vi "test TCX read (installed 71).vi"() -> ()   [LabVIEW 2011] (continued)
xmlns=\"http://www.garmin.com/xmlschemas/ActivityExtension/v2\"><Watts>208</Watts></TPX></Extensions></Trackpoint><Trackpoint><Time>2008-03-03T13:56:22Z</Time><Position><LatitudeDegrees>35.875378</LatitudeDegrees><LongitudeDegrees>-78.923548</LongitudeDegrees></Position><AltitudeMeters>77.523</AltitudeMeters><DistanceMeters>4523.565</DistanceMeters><Cadence>69</Cadence><Extensions><TPX xmlns=\"http://www.garmin.com/xmlschemas/ActivityExtension/v2\"><Watts>205</Watts></TPX></Extensions></Trackpoint><Trackpoint><Time>2008-03-03T13:56:23Z</Time><Position><LatitudeDegrees>35.875378</LatitudeDegrees><LongitudeDegrees>-78.923468</LongitudeDegrees></Position><AltitudeMeters>77.523</AltitudeMeters><DistanceMeters>4530.843</DistanceMeters><Cadence>68</Cadence><Extensions><TPX xmlns=\"http://www.garmin.com/xmlschemas/ActivityExtension/v2\"><Watts>201</Watts></TPX></Extensions></Trackpoint><Trackpoint><Time>2008-03-03T13:56:24Z</Time><Position><LatitudeDegrees>35.875380</LatitudeDegrees><LongitudeDegrees>-78.923390</LongitudeDegrees></Position><AltitudeMeters>77.523</AltitudeMeters><DistanceMeters>4537.809</DistanceMeters><Cadence>68</Cadence><Extensions><TPX xmlns=\"http://www.garmin.com/xmlschemas/ActivityExtension/v2\"><Watts>202</Watts></TPX></Extensions></Trackpoint><Trackpoint><Time>2008-03-03T13:56:25Z</Time><Position><LatitudeDegrees>35.875383</LatitudeDegrees><LongitudeDegrees>-78.923315</LongitudeDegrees></Position><AltitudeMeters>78.004</AltitudeMeters><DistanceMeters>4544.542</DistanceMeters><Cadence>68</Cadence><Extensions><TPX xmlns=\"http://www.garmin.com/xmlschemas/ActivityExtension/v2\"><Watts>207</Watts></TPX></Extensions></Trackpoint><Trackpoint><Time>2008-03-03T13:56:26Z</Time><Position><LatitudeDegrees>35.875382</LatitudeDegrees><LongitudeDegrees>-78.923243</LongitudeDegrees></Position><AltitudeMeters>78.485</AltitudeMeters><DistanceMeters>4551.062</DistanceMeters><Cadence>67</Cadence><Extensions><TPX xmlns=\"http://www.garmin.com/xmlschemas/ActivityExtension/v2\"><Watts>264</Watts></TPX></Extensions></Trackpoint><Trackpoint><Time>2008-03-03T13:56:27Z</Time><Position><LatitudeDegrees>35.875381</LatitudeDegrees><LongitudeDegrees>-78.923173</LongitudeDegrees></Position><AltitudeMeters>78.965</AltitudeMeters><DistanceMeters>4557.379</DistanceMeters><Cadence>69</Cadence><Extensions><TPX xmlns=\"http://www.garmin.com/xmlschemas/ActivityExtension/v2\"><Watts>374</Watts></TPX></Extensions></Trackpoint><Trackpoint><Time>2008-03-03T13:56:28Z</Time><Position><LatitudeDegrees>35.875390</LatitudeDegrees><LongitudeDegrees>-78.923102</LongitudeDegrees></Position><AltitudeMeters>78.965</AltitudeMeters><DistanceMeters>4563.882</DistanceMeters><Cadence>70</Cadence><Extensions><TPX xmlns=\"http://www.garmin.com/xmlschemas/ActivityExtension/v2\"><Watts>494</Watts></TPX></Extensions></Trackpoint><Trackpoint><Time>2008-03-03T13:56:29Z</Time><Position><LatitudeDegrees>35.875391</LatitudeDegrees><LongitudeDegrees>-78.923028</LongitudeDegrees></Position><AltitudeMeters>79.446</AltitudeMeters><DistanceMeters>4570.581</DistanceMeters><Cadence>70</Cadence><Extensions><TPX xmlns=\"http://www.garmin.com/xmlschemas/ActivityExtension/v2\"><Watts>505</Watts></TPX></Extensions></Trackpoint><Trackpoint><Time>2008-03-03T13:56:30Z</Time><Position><LatitudeDegrees>35.875391</LatitudeDegrees><LongitudeDegrees>-78.922954</LongitudeDegrees></Position><AltitudeMeters>80.407</AltitudeMeters><DistanceMeters>4577.208</DistanceMeters><Cadence>70</Cadence><Extensions><TPX xmlns=\"http://www.garmin.com/xmlschemas/ActivityExtension/v2\"><Watts>564</Watts></TPX></Extensions></Trackpoint><Trackpoint><Time>2008-03-03T13:56:31Z</Time><Position><LatitudeDegrees>35.875394</LatitudeDegrees><LongitudeDegrees>-78.922883</LongitudeDegrees></Position><AltitudeMeters>80.407</AltitudeMeters><DistanceMeters>4583.685</DistanceMeters><Cadence>70</Cadence><Extensions><TPX xmlns=\"http://www.garmin.com/xmlschemas/ActivityExtension/v2\"><Watts>578</Watts></TPX></Extensions></Trackpoint><Trackpoint><Time>2008-03-03T13:56:32Z</Time><Position><LatitudeDegrees>35.875403</LatitudeDegrees><LongitudeDegrees>-78.922812</LongitudeDegrees></Position><AltitudeMeters>80.888</AltitudeMeters><DistanceMeters>4590.137</DistanceMeters><Cadence>68</Cadence><Extensions><TPX xmlns=\"http://www.garmin.com/xmlschemas/ActivityExtension/v2\"><Watts>569</Watts></TPX></Extensions></Trackpoint><Trackpoint><Time>2008-03-03T13:56:33Z</Time><Position><LatitudeDegrees>35.875404</LatitudeDegrees><LongitudeDegrees>-78.922740</LongitudeDegrees></Position><AltitudeMeters>81.849</AltitudeMeters><DistanceMeters>4596.551</DistanceMeters><Cadence>67</Cadence><Extensions><TPX xmlns=\"http://www.garmin.com/xmlschemas/ActivityExtension/v2\"><Watts>513</Watts></TPX></Extensions></Trackpoint><Trackpoint><Time>2008-03-03T13:56:34Z</Time><Position><LatitudeDegrees>35.875407</LatitudeDegrees><LongitudeDegrees>-78.922669</LongitudeDegrees></Position><AltitudeMeters>82.811</AltitudeMeters><DistanceMeters>4602.985</DistanceMeters><Cadence>67</Cadence><Extensions><TPX xmlns=\"http://www.garmin.com/xmlschemas/ActivityExtension/v2\"><Watts>512</Watts></TPX></Extensions></Trackpoint><Trackpoint><Time>2008-03-03T13:56:35Z</Time><Position><LatitudeDegrees>35.875412</LatitudeDegrees><LongitudeDegrees>-78.922599</LongitudeDegrees></Position><AltitudeMeters>82.330</AltitudeMeters><DistanceMeters>4609.317</DistanceMeters><Cadence>68</Cadence><Extensions><TPX xmlns=\"http://www.garmin.com/xmlschemas/ActivityExtension/v2\"><Watts>434</Watts></TPX></Extensions></Trackpoint><Trackpoint><Time>2008-03-03T13:56:36Z</Time><Position><LatitudeDegrees>35.875413</LatitudeDegrees><LongitudeDegrees>-78.922528</LongitudeDegrees></Position><AltitudeMeters>82.811</AltitudeMeters><DistanceMeters>4615.766</DistanceMeters><Cadence>70</Cadence><Extensions><TPX xmlns=\"http://www.garmin.com/xmlschemas/ActivityExtension/v2\"><Watts>394</Watts></TPX></Extensions></Trackpoint><Trackpoint><Time>2008-03-03T13:56:37Z</Time><Position><LatitudeDegrees>35.875414</LatitudeDegrees><LongitudeDegrees>-78.922452</LongitudeDegrees></Position><AltitudeMeters>82.330</AltitudeMeters><DistanceMeters>4622.678</DistanceMeters><Cadence>72</Cadence><Extensions><TPX xmlns=\"http://www.garmin.com/xmlschemas/ActivityExtension/v2\"><Watts>358</Watts></TPX></Extensions></Trackpoint><Trackpoint><Time>2008-03-03T13:56:38Z</Time><Position><LatitudeDegrees>35.875414</LatitudeDegrees><LongitudeDegrees>-78.922373</LongitudeDegrees></Position><AltitudeMeters>82.811</AltitudeMeters><DistanceMeters>4629.848</DistanceMeters><Cadence>75</Cadence><Extensions><TPX xmlns=\"http://www.garmin.com/xmlschemas/ActivityExtension/v2\"><Watts>320</Watts></TPX></Extensions></Trackpoint><Trackpoint><Time>2008-03-03T13:56:39Z</Time><Position><LatitudeDegrees>35.875413</LatitudeDegrees><LongitudeDegrees>-78.922292</LongitudeDegrees></Position><AltitudeMeters>82.330</AltitudeMeters><DistanceMeters>4637.147</DistanceMeters><Cadence>75</Cadence><Extensions><TPX xmlns=\"http://www.garmin.com/xmlschemas/ActivityExtension/v2\"><Watts>321</Watts></TPX></Extensions></Trackpoint><Trackpoint><Time>2008-03-03T13:56:40Z</Time><Position><LatitudeDegrees>35.875414</LatitudeDegrees><LongitudeDegrees>-78.922211</LongitudeDegrees></Position><AltitudeMeters>82.330</AltitudeMeters><DistanceMeters>4644.467</DistanceMeters><Cadence>75</Cadence><Extensions><TPX xmlns=\"http://www.garmin.com/xmlschemas/ActivityExtension/v2\"><Watts>135</Watts></TPX></Extensions></Trackpoint><Trackpoint><Time>2008-03-03T13:56:41Z</Time><Position><LatitudeDegrees>35.875416</LatitudeDegrees><LongitudeDegrees>-78.922128</LongitudeDegrees></Position><AltitudeMeters>82.811</AltitudeMeters><DistanceMeters>4651.992</DistanceMeters><Cadence>69</Cadence><Extensions><TPX xmlns=\"http://www.garmin.com/xmlschemas/ActivityExtension/v2\"><Watts>125</Watts></TPX></Extensions></Trackpoint><Trackpoint><Time>2008-03-03T13:56:42Z</Time><Position><LatitudeDegrees>35.875415</LatitudeDegrees><LongitudeDegrees>-78.922042</LongitudeDegrees></Position><AltitudeMeters>82.330</AltitudeMeters><DistanceMeters>4659.760</DistanceMeters><Cadence>71</Cadence><Extensions><TPX xmlns=\"http://www.garmin.com/xmlschemas/ActivityExtension/v2\"><Watts>114</Watts></TPX></Extensions></Trackpoint><Trackpoint><Time>2008-03-03T13:56:43Z</Time><Position><LatitudeDegrees>35.875410</LatitudeDegrees><LongitudeDegrees>-78.921953</LongitudeDegrees></Position><AltitudeMeters>82.330</AltitudeMeters><DistanceMeters>4667.842</DistanceMeters><Cadence>69</Cadence><Extensions><TPX xmlns=\"http://www.garmin.com/xmlschemas/ActivityExtension/v2\"><Watts>102</Watts></TPX></Extensions></Trackpoint><Trackpoint><Time>2008-03-03T13:56:44Z</Time><Position><LatitudeDegrees>35.875404</LatitudeDegrees><LongitudeDegrees>-78.921860</LongitudeDegrees></Position><AltitudeMeters>81.849</AltitudeMeters><DistanceMeters>4676.255</DistanceMeters><Cadence>69</Cadence><Extensions><TPX xmlns=\"http://www.garmin.com/xmlschemas/ActivityExtension/v2\"><Watts>89</Watts></TPX></Extensions></Trackpoint><Trackpoint><Time>2008-03-03T13:56:45Z</Time><Position><LatitudeDegrees>35.875404</LatitudeDegrees><LongitudeDegrees>-78.921764</LongitudeDegrees></Position><AltitudeMeters>80.888</AltitudeMeters><DistanceMeters>4684.944</DistanceMeters><Cadence>67</Cadence><Extensions><TPX xmlns=\"http://www.garmin.com/xmlschemas/ActivityExtension/v2\"><Watts>90</Watts></TPX></Extensions></Trackpoint><Trackpoint><Time>2008-03-03T13:56:46Z</Time><Position><LatitudeDegrees>35.875404</LatitudeDegrees><LongitudeDegrees>-78.921664</LongitudeDegrees></Position><AltitudeMeters>80.888</AltitudeMeters><DistanceMeters>4693.956</DistanceMeters><Cadence>68</Cadence><Extensions><TPX xmlns=\"http://www.garmin.com/xmlschemas/ActivityExtension/v2\"><Watts>110</Watts></TPX></Extensions></Trackpoint><Trackpoint><Time>2008-03-03T13:56:47Z</Time><Position><LatitudeDegrees>35.875406</LatitudeDegrees><LongitudeDegrees>-78.921562</LongitudeDegrees></Position><AltitudeMeters>80.888</AltitudeMeters><DistanceMeters>4703.153</DistanceMeters><Cadence>70</Cadence><Extensions><TPX xmlns=\"http://www.garmin.com/xmlschemas/ActivityExtension/v2\"><Watts>137</Watts></TPX></Extensions></Trackpoint><Trackpoint><Time>2008-03-03T13:56:48Z</Time><Position><LatitudeDegrees>35.875412</LatitudeDegrees><LongitudeDegrees>-78.921459</LongitudeDegrees></Position><AltitudeMeters>80.407</AltitudeMeters><DistanceMeters>4712.552</DistanceMeters><Cadence>71</Cadence><Extensions><TPX xmlns=\"http://www.garmin.com/xmlschemas/ActivityExtension/v2\"><Watts>156</Watts></TPX></Extensions></Trackpoint><Trackpoint><Time>2008-03-03T13:56:49Z</Time><Position><LatitudeDegrees>35.875417</LatitudeDegrees><LongitudeDegrees>-78.921355</LongitudeDegrees></Position><AltitudeMeters>80.407</AltitudeMeters><DistanceMeters>4721.973</DistanceMeters><Cadence>71</Cadence><Extensions><TPX xmlns=\"http://www.garmin.com/xmlschemas/ActivityExtension/v2\"><Watts>177</Watts></TPX></Extensions></Trackpoint><Trackpoint><Time>2008-03-03T13:56:50Z</Time><Position><LatitudeDegrees>35.875419</LatitudeDegrees><LongitudeDegrees>-78.921249</LongitudeDegrees></Position><AltitudeMeters>79.927</AltitudeMeters><DistanceMeters>4731.501</DistanceMeters><Cadence>72</Cadence><Extensions><TPX xmlns=\"http://www.garmin.com/xmlschemas/ActivityExtension/v2\"><Watts>205</Watts></TPX></Extensions></Trackpoint><Trackpoint><Time>2008-03-03T13:56:51Z</Time><Position><LatitudeDegrees>35.875421</LatitudeDegrees><LongitudeDegrees>-78.921144</LongitudeDegrees></Position><AltitudeMeters>80.407</AltitudeMeters><DistanceMeters>4741.016</DistanceMeters><Cadence>72</Cadence><Extensions><TPX xmlns=\"http://www.garmin.com/xmlschemas/ActivityExtension/v2\"><Watts>204</Watts></TPX></Extensions></Trackpoint><Trackpoint><Time>2008-03-03T13:56:52Z</Time><Position><LatitudeDegrees>35.875422</LatitudeDegrees><LongitudeDegrees>-78.921038</LongitudeDegrees></Position><AltitudeMeters>80.407</AltitudeMeters><DistanceMeters>4750.605</DistanceMeters><Cadence>72</Cadence><Extensions><TPX xmlns=\"http://www.garmin.com/xmlschemas/ActivityExtension/v2\"><Watts>223</Watts></TPX></Extensions></Trackpoint><Trackpoint><Time>2008-03-03T13:56:53Z</Time><Position><LatitudeDegrees>35.875425</LatitudeDegrees><LongitudeDegrees>-78.920933</LongitudeDegrees></Position><AltitudeMeters>79.927</AltitudeMeters><DistanceMeters>4760.038</DistanceMeters><Cadence>72</Cadence><Extensions><TPX xmlns=\"http://www.garmin.com/xmlschemas/ActivityExtension/v2\"><Watts>226</Watts></TPX></Extensions></Trackpoint><Trackpoint><Time>2008-03-03T13:56:54Z</Time><Position><LatitudeDegrees>35.875429</LatitudeDegrees><LongitudeDegrees>-78.920829</LongitudeDegrees></Position><AltitudeMeters>80.407</AltitudeMeters><DistanceMeters>4769.412</DistanceMeters><Cadence>71</Cadence><Extensions><TPX xmlns=\"http://www.garmin.com/xmlschemas/ActivityExtension/v2\"><Watts>202</Watts></TPX></Extensions></Trackpoint><Trackpoint><Time>2008-03-03T13:56:55Z</Time><Position><LatitudeDegrees>35.875434</LatitudeDegrees><LongitudeDegrees>-78.920726</LongitudeDegrees></Position><AltitudeMeters>79.927</AltitudeMeters><DistanceMeters>4778.739</DistanceMeters><Cadence>71</Cadence><Extensions><TPX xmlns=\"http://www.garmin.com/xmlschemas/ActivityExtension/v2\"><Watts>165</Watts></TPX></Extensions></Trackpoint><Trackpoint><Time>2008-03-03T13:56:56Z</Time><Position><LatitudeDegrees>35.875437</LatitudeDegrees><LongitudeDegrees>-78.920622</LongitudeDegrees></Position><AltitudeMeters>79.927</AltitudeMeters><DistanceMeters>4788.193</DistanceMeters><Cadence>71</Cadence><Extensions><TPX xmlns=\"http://www.garmin.com/xmlschemas/ActivityExtension/v2\"><Watts>163</Watts></TPX></Extensions></Trackpoint><Trackpoint><Time>2008-03-03T13:56:57Z</Time><Position><LatitudeDegrees>35.875439</LatitudeDegrees><LongitudeDegrees>-78.920514</LongitudeDegrees></Position><AltitudeMeters>79.927</AltitudeMeters><DistanceMeters>4797.911</DistanceMeters><Cadence>74</Cadence><Extensions><TPX xmlns=\"http://www.garmin.com/xmlschemas/ActivityExtension/v2\"><Watts>116</Watts></TPX></Extensions></Trackpoint><Trackpoint><Time>2008-03-03T13:56:58Z</Time><Position><LatitudeDegrees>35.875442</LatitudeDegrees><LongitudeDegrees>-78.920403</LongitudeDegrees></Position><AltitudeMeters>78.965</AltitudeMeters><DistanceMeters>4807.962</DistanceMeters><Cadence>76</Cadence><Extensions><TPX xmlns=\"http://www.garmin.com/xmlschemas/ActivityExtension/v2\"><Watts>108</Watts></TPX></Extensions></Trackpoint><Trackpoint><Time>2008-03-03T13:56:59Z</Time><Position><LatitudeDegrees>35.875448</LatitudeDegrees><LongitudeDegrees>-78.920288</LongitudeDegrees></Position><AltitudeMeters>79.446</AltitudeMeters><DistanceMeters>4818.466</DistanceMeters><Cadence>79</Cadence><Extensions><TPX xmlns=\"http://www.garmin.com/xmlschemas/ActivityExtension/v2\"><Watts>108</Watts></TPX></Extensions></Trackpoint><Trackpoint><Time>2008-03-03T13:57:00Z</Time><Position><LatitudeDegrees>35.875454</LatitudeDegrees><LongitudeDegrees>-78.920167</LongitudeDegrees></Position><AltitudeMeters>78.485</AltitudeMeters><DistanceMeters>4829.355</DistanceMeters><Cadence>84</Cadence><Extensions><TPX xmlns=\"http://www.garmin.com/xmlschemas/ActivityExtension/v2\"><Watts>102</Watts></TPX></Extensions></Trackpoint><Trackpoint><Time>2008-03-03T13:57:01Z</Time><Position><LatitudeDegrees>35.875459</LatitudeDegrees><LongitudeDegrees>-78.920043</LongitudeDegrees></Position><AltitudeMeters>78.004</AltitudeMeters><DistanceMeters>4840.638</DistanceMeters><Cadence>85</Cadence><Extensions><TPX xmlns=\"http://www.garmin.com/xmlschemas/ActivityExtension/v2\"><Watts>100</Watts></TPX></Extensions></Trackpoint><Trackpoint><Time>2008-03-03T13:57:02Z</Time><Position><LatitudeDegrees>35.875466</LatitudeDegrees><LongitudeDegrees>-78.919916</LongitudeDegrees></Position><AltitudeMeters>77.043</AltitudeMeters><DistanceMeters>4852.169</DistanceMeters><Cadence>87</Cadence><Extensions><TPX xmlns=\"http://www.garmin.com/xmlschemas/ActivityExtension/v2\"><Watts>102</Watts></TPX></Extensions></Trackpoint><Trackpoint><Time>2008-03-03T13:57:03Z</Time><Position><LatitudeDegrees>35.875471</LatitudeDegrees><LongitudeDegrees>-78.919786</LongitudeDegrees></Position><AltitudeMeters>76.562</AltitudeMeters><DistanceMeters>4863.915</DistanceMeters><Cadence>89</Cadence><Extensions><TPX xmlns=\"http://www.garmin.com/xmlschemas/ActivityExtension/v2\"><Watts>106</Watts></TPX></Extensions></Trackpoint><Trackpoint><Time>2008-03-03T13:57:04Z</Time><Position><LatitudeDegrees>35.875501</LatitudeDegrees><LongitudeDegrees>-78.919659</LongitudeDegrees></Position><AltitudeMeters>76.562</AltitudeMeters><DistanceMeters>4875.472</DistanceMeters><Cadence>90</Cadence><Extensions><TPX xmlns=\"http://www.garmin.com/xmlschemas/ActivityExtension/v2\"><Watts>120</Watts></TPX></Extensions></Trackpoint><Trackpoint><Time>2008-03-03T13:57:05Z</Time><Position><LatitudeDegrees>35.875514</LatitudeDegrees><LongitudeDegrees>-78.919528</LongitudeDegrees></Position><AltitudeMeters>76.562</AltitudeMeters><DistanceMeters>4887.392</DistanceMeters><Cadence>92</Cadence><Extensions><TPX xmlns=\"http://www.garmin.com/xmlschemas/ActivityExtension/v2\"><Watts>196</Watts></TPX></Extensions></Trackpoint><Trackpoint><Time>2008-03-03T13:57:06Z</Time><Position><LatitudeDegrees>35.875526</LatitudeDegrees><LongitudeDegrees>-78.919395</LongitudeDegrees></Position><AltitudeMeters>75.120</AltitudeMeters><DistanceMeters>4899.475</DistanceMeters><Cadence>92</Cadence><Extensions><TPX xmlns=\"http://www.garmin.com/xmlschemas/ActivityExtension/v2\"><Watts>194</Watts></TPX></Extensions></Trackpoint><Trackpoint><Time>2008-03-03T13:57:07Z</Time><Position><LatitudeDegrees>35.875539</LatitudeDegrees><LongitudeDegrees>-78.919260</LongitudeDegrees></Position><AltitudeMeters>74.640</AltitudeMeters><DistanceMeters>4911.710</DistanceMeters><Cadence>92</Cadence><Extensions><TPX xmlns=\"http://www.garmin.com/xmlschemas/ActivityExtension/v2\"><Watts>168</Watts></TPX></Extensions></Trackpoint><Trackpoint><Time>2008-03-03T13:57:08Z</Time><Position><LatitudeDegrees>35.875557</LatitudeDegrees><LongitudeDegrees>-78.919127</LongitudeDegrees></Position><AltitudeMeters>75.120</AltitudeMeters><DistanceMeters>4923.924</DistanceMeters><Cadence>92</Cadence><Extensions><TPX xmlns=\"http://www.garmin.com/xmlschemas/ActivityExtension/v2\"><Watts>167</Watts></TPX></Extensions></Trackpoint><Trackpoint><Time>2008-03-03T13:57:09Z</Time><Position><LatitudeDegrees>35.875570</LatitudeDegrees><LongitudeDegrees>-78.918995</LongitudeDegrees></Position><AltitudeMeters>74.640</AltitudeMeters><DistanceMeters>4935.932</DistanceMeters><Cadence>91</Cadence><Extensions><TPX xmlns=\"http://www.garmin.com/xmlschemas/ActivityExtension/v2\"><Watts>131</Watts></TPX></Extensions></Trackpoint><Trackpoint><Time>2008-03-03T13:57:10Z</Time><Position><LatitudeDegrees>35.875582</LatitudeDegrees><LongitudeDegrees>-78.918863</LongitudeDegrees></Position><AltitudeMeters>74.159</AltitudeMeters><DistanceMeters>4947.869</DistanceMeters><Cadence>90</Cadence><Extensions><TPX xmlns=\"http://www.garmin.com/xmlschemas/ActivityExtension/v2\"><Watts>131</Watts></TPX></Extensions></Trackpoint><Trackpoint><Time>2008-03-03T13:57:11Z</Time><Position><LatitudeDegrees>35.875593</LatitudeDegrees><LongitudeDegrees>-78.918733</LongitudeDegrees></Position><AltitudeMeters>74.159</AltitudeMeters><DistanceMeters>4959.708</DistanceMeters><Cadence>90</Cadence><Extensions><TPX xmlns=\"http://www.garmin.com/xmlschemas/ActivityExtension/v2\"><Watts>133</Watts></TPX></Extensions></Trackpoint><Trackpoint><Time>2008-03-03T13:57:12Z</Time><Position><LatitudeDegrees>35.875601</LatitudeDegrees><LongitudeDegrees>-78.918603</LongitudeDegrees></Position><AltitudeMeters>73.678</AltitudeMeters><DistanceMeters>4971.460</DistanceMeters><Cadence>89</Cadence><Extensions><TPX xmlns=\"http://www.garmin.com/xmlschemas/ActivityExtension/v2\"><Watts>119</Watts></TPX></Extensions></Trackpoint><Trackpoint><Time>2008-03-03T13:57:13Z</Time><Position><LatitudeDegrees>35.875612</LatitudeDegrees><LongitudeDegrees>-78.918475</LongitudeDegrees></Position><AltitudeMeters>72.717</AltitudeMeters><DistanceMeters>4983.142</DistanceMeters><Cadence>88</Cadence><Extensions><TPX xmlns=\"http://www.garmin.com/xmlschemas/ActivityExtension/v2\"><Watts>119</Watts></TPX></Extensions></Trackpoint><Trackpoint><Time>2008-03-03T13:57:14Z</Time><Position><LatitudeDegrees>35.875627</LatitudeDegrees><LongitudeDegrees>-78.918347</LongitudeDegrees></Position><AltitudeMeters>73.198</AltitudeMeters><DistanceMeters>4994.779</DistanceMeters><Cadence>88</Cadence><Extensions><TPX xmlns=\"http://www.garmin.com/xmlschemas/ActivityExtension/v2\"><Watts>124</Watts></TPX></Extensions></Trackpoint><Trackpoint><Time>2008-03-03T13:57:15Z</Time><Position><LatitudeDegrees>35.875641</LatitudeDegrees><LongitudeDegrees>-78.918221</LongitudeDegrees></Position><AltitudeMeters>72.717</AltitudeMeters><DistanceMeters>5006.281</DistanceMeters><Cadence>87</Cadence><Extensions><TPX xmlns=\"http://www.garmin.com/xmlschemas/ActivityExtension/v2\"><Watts>152</Watts></TPX></Extensions></Trackpoint><Trackpoint><Time>2008-03-03T13:57:16Z</Time><Position><LatitudeDegrees>35.875651</LatitudeDegrees><LongitudeDegrees>-78.918096</LongitudeDegrees></Position><AltitudeMeters>72.236</AltitudeMeters><DistanceMeters>5017.583</DistanceMeters><Cadence>87</Cadence><Extensions><TPX xmlns=\"http://www.garmin.com/xmlschemas/ActivityExtension/v2\"><Watts>151</Watts></TPX></Extensions></Trackpoint><Trackpoint><Time>2008-03-03T13:57:17Z</Time><Position><LatitudeDegrees>35.875662</LatitudeDegrees><LongitudeDegrees>-78.917972</LongitudeDegrees></Position><AltitudeMeters>72.717</AltitudeMeters><DistanceMeters>5028.809</DistanceMeters><Cadence>85</Cadence><Extensions><TPX xmlns=\"http://www.garmin.com/xmlschemas/ActivityExtension/v2\"><Watts>171</Watts></TPX></Extensions></Trackpoint><Trackpoint><Time>2008-03-03T13:57:18Z</Time><Position><LatitudeDegrees>35.875675</LatitudeDegrees><LongitudeDegrees>-78.917850</LongitudeDegrees></Position><AltitudeMeters>72.236</AltitudeMeters><DistanceMeters>5039.949</DistanceMeters><Cadence>85</Cadence><Extensions><TPX xmlns=\"http://www.garmin.com/xmlschemas/ActivityExtension/v2\"><Watts>159</Watts></TPX></Extensions></Trackpoint><Trackpoint><Time>2008-03-03T13:57:19Z</Time><Position><LatitudeDegrees>35.875687</LatitudeDegrees><LongitudeDegrees>-78.917731</LongitudeDegrees></Position><AltitudeMeters>72.236</AltitudeMeters><DistanceMeters>5050.769</DistanceMeters><Cadence>83</Cadence><Extensions><TPX xmlns=\"http://www.garmin.com/xmlschemas/ActivityExtension/v2\"><Watts>162</Watts></TPX></Extensions></Trackpoint><Trackpoint><Time>2008-03-03T13:57:20Z</Time><Position><LatitudeDegrees>35.875697</LatitudeDegrees><LongitudeDegrees>-78.917611</LongitudeDegrees></Position><AltitudeMeters>72.236</AltitudeMeters><DistanceMeters>5061.608</DistanceMeters><Cadence>83</Cadence><Extensions><TPX xmlns=\"http://www.garmin.com/xmlschemas/ActivityExtension/v2\"><Watts>160</Watts></TPX></Extensions></Trackpoint><Trackpoint><Time>2008-03-03T13:57:21Z</Time><Position><LatitudeDegrees>35.875713</LatitudeDegrees><LongitudeDegrees>-78.917491</LongitudeDegrees></Position><AltitudeMeters>71.755</AltitudeMeters><DistanceMeters>5072.610</DistanceMeters><Cadence>83</Cadence><Extensions><TPX xmlns=\"http://www.garmin.com/xmlschemas/ActivityExtension/v2\"><Watts>191</Watts></TPX></Extensions></Trackpoint><Trackpoint><Time>2008-03-03T13:57:22Z</Time><Position><LatitudeDegrees>35.875728</LatitudeDegrees><LongitudeDegrees>-78.917372</LongitudeDegrees></Position><AltitudeMeters>71.755</AltitudeMeters><DistanceMeters>5083.461</DistanceMeters><Cadence>83</Cadence><Extensions><TPX xmlns=\"http://www.garmin.com/xmlschemas/ActivityExtension/v2\"><Watts>215</Watts></TPX></Extensions></Trackpoint><Trackpoint><Time>2008-03-03T13:57:23Z</Time><Position><LatitudeDegrees>35.875742</LatitudeDegrees><LongitudeDegrees>-78.917254</LongitudeDegrees></Position><AltitudeMeters>71.755</AltitudeMeters><DistanceMeters>5094.283</DistanceMeters><Cadence>82</Cadence><Extensions><TPX xmlns=\"http://www.garmin.com/xmlschemas/ActivityExtension/v2\"><Watts>219</Watts></TPX></Extensions></Trackpoint><Trackpoint><Time>2008-03-03T13:57:24Z</Time><Position><LatitudeDegrees>35.875754</LatitudeDegrees><LongitudeDegrees>-78.917136</LongitudeDegrees></Position><AltitudeMeters>72.236</AltitudeMeters><DistanceMeters>5105.024</DistanceMeters><Cadence>82</Cadence><Extensions><TPX xmlns=\"http://www.garmin.com/xmlschemas/ActivityExtension/v2\"><Watts>227</Watts></TPX></Extensions></Trackpoint><Trackpoint><Time>2008-03-03T13:57:25Z</Time><Position><LatitudeDegrees>35.875763</LatitudeDegrees><LongitudeDegrees>-78.917019</LongitudeDegrees></Position><AltitudeMeters>71.755</AltitudeMeters><DistanceMeters>5115.571</DistanceMeters><Cadence>80</Cadence><Extensions><TPX xmlns=\"http://www.garmin.com/xmlschemas/ActivityExtension/v2\"><Watts>226</Watts></TPX></Extensions></Trackpoint><Trackpoint><Time>2008-03-03T13:57:26Z</Time><Position><LatitudeDegrees>35.875774</LatitudeDegrees><LongitudeDegrees>-78.916904</LongitudeDegrees></Position><AltitudeMeters>71.755</AltitudeMeters><DistanceMeters>5125.976</DistanceMeters><Cadence>79</Cadence><Extensions><TPX xmlns=\"http://www.garmin.com/xmlschemas/ActivityExtension/v2\"><Watts>249</Watts></TPX></Extensions></Trackpoint><Trackpoint><Time>2008-03-03T13:57:27Z</Time><Position><LatitudeDegrees>35.875782</LatitudeDegrees><LongitudeDegrees>-78.916791</LongitudeDegrees></Position><AltitudeMeters>72.236</AltitudeMeters><DistanceMeters>5136.285</DistanceMeters><Cadence>78</Cadence><Extensions><TPX xmlns=\"http://www.garmin.com/xmlschemas/ActivityExtension/v2\"><Watts>261</Watts></TPX></Extensions></Trackpoint><Trackpoint><Time>2008-03-03T13:57:28Z</Time><Position><LatitudeDegrees>35.875791</LatitudeDegrees><LongitudeDegrees>-78.916679</LongitudeDegrees></Position><AltitudeMeters>72.236</AltitudeMeters><DistanceMeters>5146.463</DistanceMeters><Cadence>77</Cadence><Extensions><TPX xmlns=\"http://www.garmin.com/xmlschemas/ActivityExtension/v2\"><Watts>269</Watts></TPX></Extensions></Trackpoint><Trackpoint><Time>2008-03-03T13:57:29Z</Time><Position><LatitudeDegrees>35.875800</LatitudeDegrees><LongitudeDegrees>-78.916569</LongitudeDegrees></Position><AltitudeMeters>71.755</AltitudeMeters><DistanceMeters>5156.314</DistanceMeters><Cadence>76</Cadence><Extensions><TPX xmlns=\"http://www.garmin.com/xmlschemas/ActivityExtension/v2\"><Watts>262</Watts></TPX></Extensions></Trackpoint><Trackpoint><Time>2008-03-03T13:57:30Z</Time><Position><LatitudeDegrees>35.875807</LatitudeDegrees><LongitudeDegrees>-78.916461</LongitudeDegrees></Position><AltitudeMeters>72.236</AltitudeMeters><DistanceMeters>5166.121</DistanceMeters><Cadence>75</Cadence><Extensions><TPX xmlns=\"http://www.garmin.com/xmlschemas/ActivityExtension/v2\"><Watts>258</Watts></TPX></Extensions></Trackpoint><Trackpoint><Time>2008-03-03T13:57:31Z</Time><Position><LatitudeDegrees>35.875811</LatitudeDegrees><LongitudeDegrees>-78.916353</LongitudeDegrees></Position><AltitudeMeters>72.236</AltitudeMeters><DistanceMeters>5175.855</DistanceMeters><Cadence>74</Cadence><Extensions><TPX xmlns=\"http://www.garmin.com/xmlschemas/ActivityExtension/v2\"><Watts>255</Watts></TPX></Extensions></Trackpoint><Trackpoint><Time>2008-03-03T13:57:32Z</Time><Position><LatitudeDegrees>35.875821</LatitudeDegrees><LongitudeDegrees>-78.916247</LongitudeDegrees></Position><AltitudeMeters>72.717</AltitudeMeters><DistanceMeters>5185.500</DistanceMeters><Cadence>73</Cadence><Extensions><TPX xmlns=\"http://www.garmin.com/xmlschemas/ActivityExtension/v2\"><Watts>252</Watts></TPX></Extensions></Trackpoint><Trackpoint><Time>2008-03-03T13:57:33Z</Time><Position><LatitudeDegrees>35.875826</LatitudeDegrees><LongitudeDegrees>-78.916141</LongitudeDegrees></Position><AltitudeMeters>72.717</AltitudeMeters><DistanceMeters>5195.045</DistanceMeters><Cadence>73</Cadence><Extensions><TPX xmlns=\"http://www.garmin.com/xmlschemas/ActivityExtension/v2\"><Watts>253</Watts></TPX></Extensions></Trackpoint><Trackpoint><Time>2008-03-03T13:57:34Z</Time><Position><LatitudeDegrees>35.875832</LatitudeDegrees><LongitudeDegrees>-78.916038</LongitudeDegrees></Position><AltitudeMeters>72.717</AltitudeMeters><DistanceMeters>5204.398</DistanceMeters><Cadence>71</Cadence><Extensions><TPX xmlns=\"http://www.garmin.com/xmlschemas/ActivityExtension/v2\"><Watts>250</Watts></TPX></Extensions></Trackpoint><Trackpoint><Time>2008-03-03T13:57:35Z</Time><Position><LatitudeDegrees>35.875837</LatitudeDegrees><LongitudeDegrees>-78.915935</LongitudeDegrees></Position><AltitudeMeters>72.717</AltitudeMeters><DistanceMeters>5213.658</DistanceMeters><Cadence>71</Cadence><Extensions><TPX xmlns=\"http://www.garmin.com/xmlschemas/ActivityExtension/v2\"><Watts>247</Watts></TPX></Extensions></Trackpoint><Trackpoint><Time>2008-03-03T13:57:36Z</Time><Position><LatitudeDegrees>35.875846</LatitudeDegrees><LongitudeDegrees>-78.915834</LongitudeDegrees></Position><AltitudeMeters>72.236</AltitudeMeters><DistanceMeters>5222.896</DistanceMeters><Cadence>71</Cadence><Extensions><TPX xmlns=\"http://www.garmin.com/xmlschemas/ActivityExtension/v2\"><Watts>243</Watts></TPX></Extensions></Trackpoint><Trackpoint><Time>2008-03-03T13:57:37Z</Time><Position><LatitudeDegrees>35.875856</LatitudeDegrees><LongitudeDegrees>-78.915733</LongitudeDegrees></Position><AltitudeMeters>72.717</AltitudeMeters><DistanceMeters>5232.086</DistanceMeters><Cadence>70</Cadence><Extensions><TPX xmlns=\"http://www.garmin.com/xmlschemas/ActivityExtension/v2\"><Watts>238</Watts></TPX></Extensions></Trackpoint><Trackpoint><Time>2008-03-03T13:57:38Z</Time><Position><LatitudeDegrees>35.875862</LatitudeDegrees><LongitudeDegrees>-78.915632</LongitudeDegrees></Position><AltitudeMeters>72.717</AltitudeMeters><DistanceMeters>5241.232</DistanceMeters><Cadence>70</Cadence><Extensions><TPX xmlns=\"http://www.garmin.com/xmlschemas/ActivityExtension/v2\"><Watts>237</Watts></TPX></Extensions></Trackpoint><Trackpoint><Time>2008-03-03T13:57:39Z</Time><Position><LatitudeDegrees>35.875868</LatitudeDegrees><LongitudeDegrees>-78.915532</LongitudeDegrees></Position><AltitudeMeters>72.236</AltitudeMeters><DistanceMeters>5250.275</DistanceMeters><Cadence>70</Cadence><Extensions><TPX xmlns=\"http://www.garmin.com/xmlschemas/ActivityExtension/v2\"><Watts>236</Watts></TPX></Extensions></Trackpoint><Trackpoint><Time>2008-03-03T13:57:40Z</Time><Position><LatitudeDegrees>35.875874</LatitudeDegrees><LongitudeDegrees>-78.915432</LongitudeDegrees></Position><AltitudeMeters>72.717</AltitudeMeters><DistanceMeters>5259.338</DistanceMeters><Cadence>69</Cadence><Extensions><TPX xmlns=\"http://www.garmin.com/xmlschemas/ActivityExtension/v2\"><Watts>224</Watts></TPX></Extensions></Trackpoint><Trackpoint><Time>2008-03-03T13:57:41Z</Time><Position><LatitudeDegrees>35.875881</LatitudeDegrees><LongitudeDegrees>-78.915332</LongitudeDegrees></Position><AltitudeMeters>72.717</AltitudeMeters><DistanceMeters>5268.324</DistanceMeters><Cadence>68</Cadence><Extensions><TPX xmlns=\"http://www.garmin.com/xmlschemas/ActivityExtension/v2\"><Watts>194</Watts></TPX></Extensions></Trackpoint><Trackpoint><Time>2008-03-03T13:57:42Z</Time><Position><LatitudeDegrees>35.875887</LatitudeDegrees><LongitudeDegrees>-78.915235</LongitudeDegrees></Position><AltitudeMeters>72.717</AltitudeMeters><DistanceMeters>5277.131</DistanceMeters><Cadence>66</Cadence><Extensions><TPX xmlns=\"http://www.garmin.com/xmlschemas/ActivityExtension/v2\"><Watts>128</Watts></TPX></Extensions></Trackpoint><Trackpoint><Time>2008-03-03T13:57:43Z</Time><Position><LatitudeDegrees>35.875895</LatitudeDegrees><LongitudeDegrees>-78.915140</LongitudeDegrees></Position><AltitudeMeters>73.198</AltitudeMeters><DistanceMeters>5285.762</DistanceMeters><Cadence>66</Cadence><Extensions><TPX xmlns=\"http://www.garmin.com/xmlschemas/ActivityExtension/v2\"><Watts>136</Watts></TPX></Extensions></Trackpoint><Trackpoint><Time>2008-03-03T13:57:44Z</Time><Position><LatitudeDegrees>35.875906</LatitudeDegrees><LongitudeDegrees>-78.915048</LongitudeDegrees></Position><AltitudeMeters>73.198</AltitudeMeters><DistanceMeters>5294.190</DistanceMeters><Cadence>63</Cadence><Extensions><TPX xmlns=\"http://www.garmin.com/xmlschemas/ActivityExtension/v2\"><Watts>103</Watts></TPX></Extensions></Trackpoint><Trackpoint><Time>2008-03-03T13:57:45Z</Time><Position><LatitudeDegrees>35.875911</LatitudeDegrees><LongitudeDegrees>-78.914957</LongitudeDegrees></Position><AltitudeMeters>73.198</AltitudeMeters><DistanceMeters>5302.393</DistanceMeters><Cadence>63</Cadence><Extensions><TPX xmlns=\"http://www.garmin.com/xmlschemas/ActivityExtension/v2\"><Watts>102</Watts></TPX></Extensions></Trackpoint><Trackpoint><Time>2008-03-03T13:57:46Z</Time><Position><LatitudeDegrees>35.875901</LatitudeDegrees><LongitudeDegrees>-78.914872</LongitudeDegrees></Position><AltitudeMeters>73.198</AltitudeMeters><DistanceMeters>5310.137</DistanceMeters><Cadence>61</Cadence><Extensions><TPX xmlns=\"http://www.garmin.com/xmlschemas/ActivityExtension/v2\"><Watts>101</Watts></TPX></Extensions></Trackpoint><Trackpoint><Time>2008-03-03T13:57:47Z</Time><Position><LatitudeDegrees>35.875843</LatitudeDegrees><LongitudeDegrees>-78.914815</LongitudeDegrees></Position><AltitudeMeters>72.717</AltitudeMeters><DistanceMeters>5318.377</DistanceMeters><Cadence>60</Cadence><Extensions><TPX xmlns=\"http://www.garmin.com/xmlschemas/ActivityExtension/v2\"><Watts>100</Watts></TPX></Extensions></Trackpoint><Trackpoint><Time>2008-03-03T13:57:48Z</Time><Position><LatitudeDegrees>35.875778</LatitudeDegrees><LongitudeDegrees>-78.914785</LongitudeDegrees></Position><AltitudeMeters>73.198</AltitudeMeters><DistanceMeters>5326.127</DistanceMeters><Cadence>60</Cadence><Extensions><TPX xmlns=\"http://www.garmin.com/xmlschemas/ActivityExtension/v2\"><Watts>101</Watts></TPX></Extensions></Trackpoint><Trackpoint><Time>2008-03-03T13:57:49Z</Time><Position><LatitudeDegrees>35.875707</LatitudeDegrees><LongitudeDegrees>-78.914769</LongitudeDegrees></Position><AltitudeMeters>73.198</AltitudeMeters><DistanceMeters>5334.156</DistanceMeters><Cadence>60</Cadence><Extensions><TPX xmlns=\"http://www.garmin.com/xmlschemas/ActivityExtension/v2\"><Watts>197</Watts></TPX></Extensions></Trackpoint><Trackpoint><Time>2008-03-03T13:57:50Z</Time><Position><LatitudeDegrees>35.875634</LatitudeDegrees><LongitudeDegrees>-78.914751</LongitudeDegrees></Position><AltitudeMeters>73.198</AltitudeMeters><DistanceMeters>5342.338</DistanceMeters><Cadence>62</Cadence><Extensions><TPX xmlns=\"http://www.garmin.com/xmlschemas/ActivityExtension/v2\"><Watts>233</Watts></TPX></Extensions></Trackpoint><Trackpoint><Time>2008-03-03T13:57:51Z</Time><Position><LatitudeDegrees>35.875561</LatitudeDegrees><LongitudeDegrees>-78.914726</LongitudeDegrees></Position><AltitudeMeters>72.717</AltitudeMeters><DistanceMeters>5350.732</DistanceMeters><Cadence>63</Cadence><Extensions><TPX xmlns=\"http://www.garmin.com/xmlschemas/ActivityExtension/v2\"><Watts>244</Watts></TPX></Extensions></Trackpoint><Trackpoint><Time>2008-03-03T13:57:52Z</Time><Position><LatitudeDegrees>35.875487</LatitudeDegrees><LongitudeDegrees>-78.914696</LongitudeDegrees></Position><AltitudeMeters>72.717</AltitudeMeters><DistanceMeters>5359.455</DistanceMeters><Cadence>64</Cadence><Extensions><TPX xmlns=\"http://www.garmin.com/xmlschemas/ActivityExtension/v2\"><Watts>245</Watts></TPX></Extensions></Trackpoint><Trackpoint><Time>2008-03-03T13:57:53Z</Time><Position><LatitudeDegrees>35.875409</LatitudeDegrees><LongitudeDegrees>-78.914659</LongitudeDegrees></Position><AltitudeMeters>73.198</AltitudeMeters><DistanceMeters>5368.707</DistanceMeters><Cadence>65</Cadence><Extensions><TPX xmlns=\"http://www.garmin.com/xmlschemas/ActivityExtension/v2\"><Watts>247</Watts></TPX></Extensions></Trackpoint><Trackpoint><Time>2008-03-03T13:57:54Z</Time><Position><LatitudeDegrees>35.875334</LatitudeDegrees><LongitudeDegrees>-78.914618</LongitudeDegrees></Position><AltitudeMeters>73.198</AltitudeMeters><DistanceMeters>5377.795</DistanceMeters><Cadence>66</Cadence><Extensions><TPX xmlns=\"http://www.garmin.com/xmlschemas/ActivityExtension/v2\"><Watts>241</Watts></TPX></Extensions></Trackpoint><Trackpoint><Time>2008-03-03T13:57:55Z</Time><Position><LatitudeDegrees>35.875254</LatitudeDegrees><LongitudeDegrees>-78.914572</LongitudeDegrees></Position><AltitudeMeters>72.717</AltitudeMeters><DistanceMeters>5387.640</DistanceMeters><Cadence>66</Cadence><Extensions><TPX xmlns=\"http://www.garmin.com/xmlschemas/ActivityExtension/v2\"><Watts>217</Watts></TPX></Extensions></Trackpoint><Trackpoint><Time>2008-03-03T13:57:56Z</Time><Position><LatitudeDegrees>35.875181</LatitudeDegrees><LongitudeDegrees>-78.914526</LongitudeDegrees></Position><AltitudeMeters>72.717</AltitudeMeters><DistanceMeters>5396.782</DistanceMeters><Cadence>67</Cadence><Extensions><TPX xmlns=\"http://www.garmin.com/xmlschemas/ActivityExtension/v2\"><Watts>210</Watts></TPX></Extensions></Trackpoint><Trackpoint><Time>2008-03-03T13:57:57Z</Time><Position><LatitudeDegrees>35.875107</LatitudeDegrees><LongitudeDegrees>-78.914479</LongitudeDegrees></Position><AltitudeMeters>72.717</AltitudeMeters><DistanceMeters>5405.918</DistanceMeters><Cadence>68</Cadence><Extensions><TPX xmlns=\"http://www.garmin.com/xmlschemas/ActivityExtension/v2\"><Watts>194</Watts></TPX></Extensions></Trackpoint><Trackpoint><Time>2008-03-03T13:57:58Z</Time><Position><LatitudeDegrees>35.875018</LatitudeDegrees><LongitudeDegrees>-78.914426</LongitudeDegrees></Position><AltitudeMeters>72.717</AltitudeMeters><DistanceMeters>5416.953</DistanceMeters><Cadence>68</Cadence><Extensions><TPX xmlns=\"http://www.garmin.com/xmlschemas/ActivityExtension/v2\"><Watts>172</Watts></TPX></Extensions></Trackpoint><Trackpoint><Time>2008-03-03T13:57:59Z</Time><Position><LatitudeDegrees>35.874941</LatitudeDegrees><LongitudeDegrees>-78.914381</LongitudeDegrees></Position><AltitudeMeters>72.717</AltitudeMeters><DistanceMeters>5426.388</DistanceMeters><Cadence>69</Cadence><Extensions><TPX xmlns=\"http://www.garmin.com/xmlschemas/ActivityExtension/v2\"><Watts>169</Watts></TPX></Extensions></Trackpoint><Trackpoint><Time>2008-03-03T13:58:00Z</Time><Position><LatitudeDegrees>35.874859</LatitudeDegrees><LongitudeDegrees>-78.914330</LongitudeDegrees></Position><AltitudeMeters>72.717</AltitudeMeters><DistanceMeters>5436.635</DistanceMeters><Cadence>69</Cadence><Extensions><TPX xmlns=\"http://www.garmin.com/xmlschemas/ActivityExtension/v2\"><Watts>168</Watts></TPX></Extensions></Trackpoint><Trackpoint><Time>2008-03-03T13:58:01Z</Time><Position><LatitudeDegrees>35.874782</LatitudeDegrees><LongitudeDegrees>-78.914282</LongitudeDegrees></Position><AltitudeMeters>72.717</AltitudeMeters><DistanceMeters>5446.125</DistanceMeters><Cadence>69</Cadence><Extensions><TPX xmlns=\"http://www.garmin.com/xmlschemas/ActivityExtension/v2\"><Watts>165</Watts></TPX></Extensions></Trackpoint><Trackpoint><Time>2008-03-03T13:58:02Z</Time><Position><LatitudeDegrees>35.874708</LatitudeDegrees><LongitudeDegrees>-78.914236</LongitudeDegrees></Position><AltitudeMeters>72.717</AltitudeMeters><DistanceMeters>5455.360</DistanceMeters><Cadence>69</Cadence><Extensions><TPX xmlns=\"http://www.garmin.com/xmlschemas/ActivityExtension/v2\"><Watts>160</Watts></TPX></Extensions></Trackpoint><Trackpoint><Time>2008-03-03T13:58:03Z</Time><Position><LatitudeDegrees>35.874639</LatitudeDegrees><LongitudeDegrees>-78.914188</LongitudeDegrees></Position><AltitudeMeters>72.717</AltitudeMeters><DistanceMeters>5464.177</DistanceMeters><Cadence>70</Cadence><Extensions><TPX xmlns=\"http://www.garmin.com/xmlschemas/ActivityExtension/v2\"><Watts>159</Watts></TPX></Extensions></Trackpoint><Trackpoint><Time>2008-03-03T13:58:04Z</Time><Position><LatitudeDegrees>35.874564</LatitudeDegrees><LongitudeDegrees>-78.914139</LongitudeDegrees></
